vi "my_graph_parabola.vi"() -> ()   [LabVIEW 2019]
uses:
  <vilib>/Analysis/1siggen.llb/Ramp Pattern by Delta.vi
  <vilib>/Analysis/NI_AALBase.lvlib
panel:
  out "y_point":dbl
  in  "x_point":dbl(slide) scale=-2.0..2.0
  in  "stop":bool
  in  "x_start":dbl=-2.0
  in  "x_end":dbl=2.0
  in  "x_delta":dbl=0.001
  in  "c":dbl
  in  "b":dbl
  in  "a":dbl
  out "XY Graph":cluster{"Ramp Pattern":dbl[], dbl[]}[](graph)
  # "a"
  # "b"
  # "c"
  # "y"
  # "x"
  # "y=a*x*x+b*x+c"
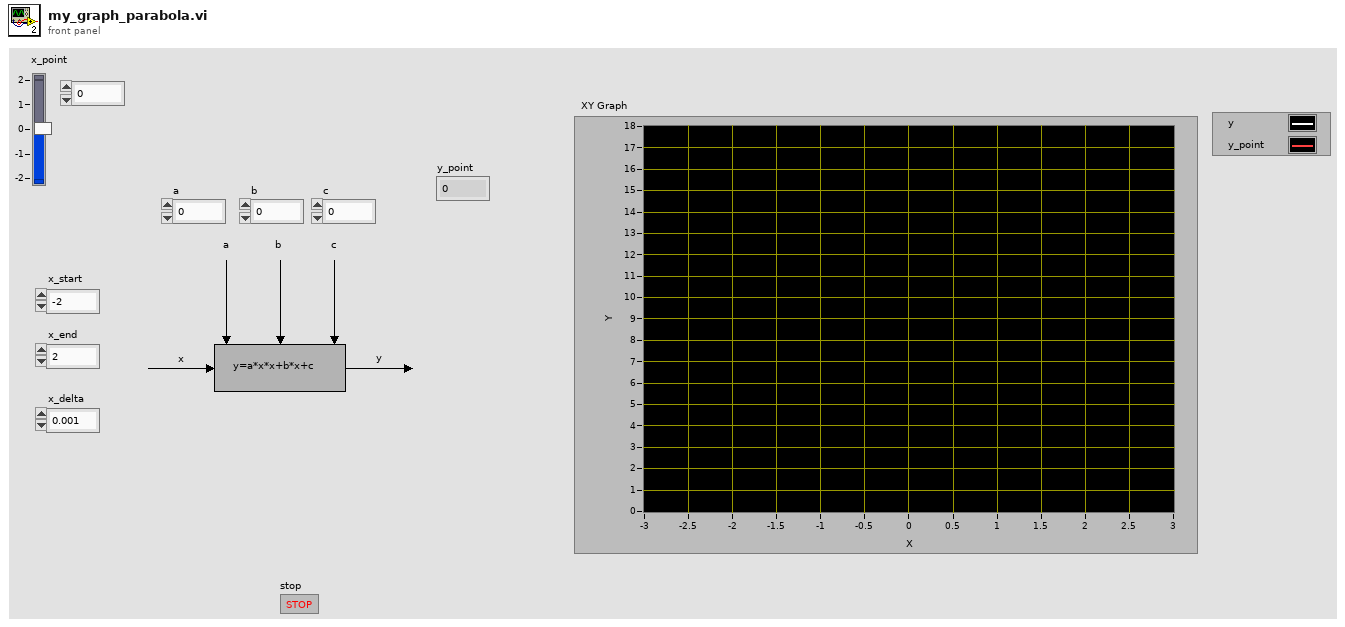
[diagram p1: front panel]
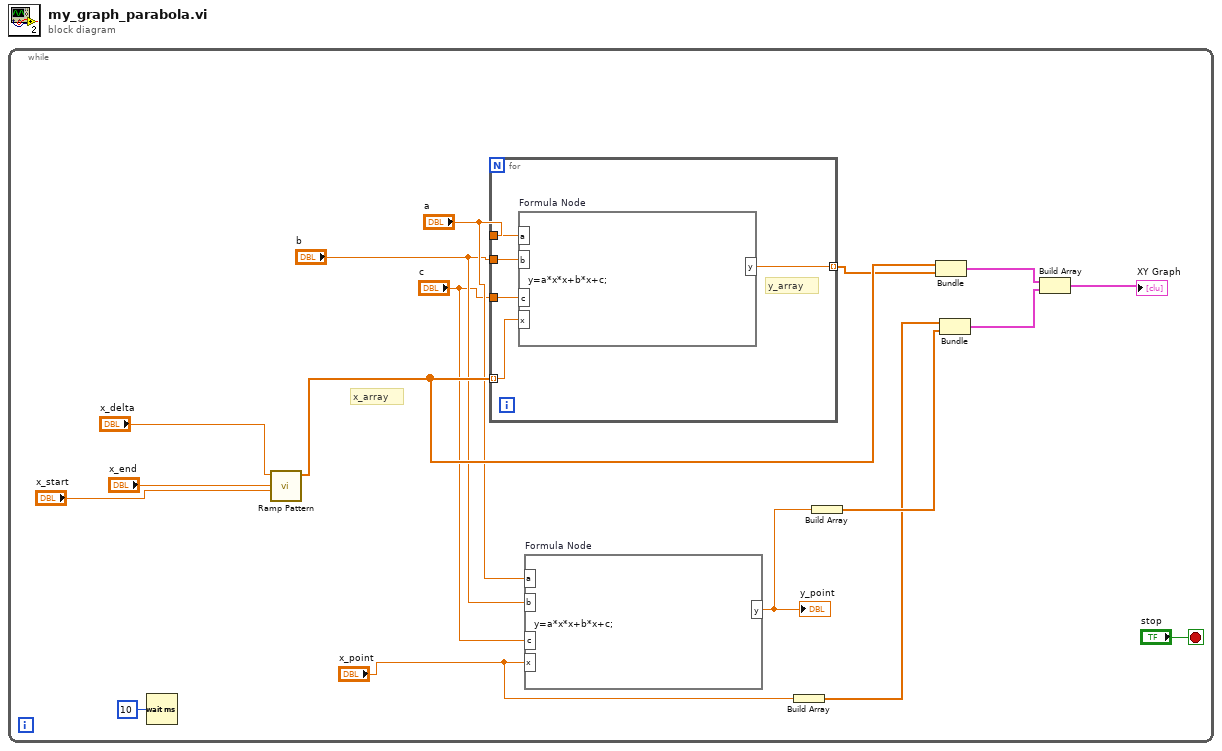
[diagram p0: block diagram]
diagram:
  n1 = while {
    stop <- "stop" stop-if-true
    # "x_array"
    n2 = Wait (ms)(milliseconds to wait=u32 10) -> ()  [unwired: 1 out]
    n3 = call-poly <vilib>:"Ramp Pattern.vi"("start"="x_start", "end"="x_end", "delta"="x_delta") -> ("Ramp Pattern"=w17:dbl[])  [unwired: 6 in, 2 out]
    n4 = for {
      tunnel: "a" -> [w22]
      tunnel: "b" -> [w21]
      tunnel: "c" -> [w20]
      tunnel: w17 -> [w19] mode=indexing
      tunnel: [w18] -> w16 mode=indexing
      # "y_array"
      n5 = formula code="y=a*x*x+b*x+c;"("a"=w22, "b"=w21, "c"=w20, "x"=w19) -> ("y"=w18:dbl)
    }
    n6 = formula code="y=a*x*x+b*x+c;"("a"="a", "b"="b", "c"="c", "x"="x_point") -> ("y"=w3:dbl)
    "y_point" <- w3
    n7 = Build Array("x_point") -> (w1:dbl[])
    n8 = Build Array(w3) -> (w2:dbl[])
    n9 = Bundle "Bundle"("Ramp Pattern"=w17, w16) -> (w10:cluster{"Ramp Pattern":dbl[], dbl[]})  [unwired: 1 in]
    n10 = Bundle "Bundle"(w1, w2) -> (w9:cluster{dbl[], dbl[]})  [unwired: 1 in]
    n11 = Build Array "Build Array"(w10, w9) -> (→"XY Graph":cluster{"Ramp Pattern":dbl[], dbl[]}[])
  }
